vi "_API_BINANCE_POST_DisableFastWithdrawSwich.vi"(0 "BinanceAPI in":refnum<class "BinanceAPI_.lvclass">, 11 "error in (no error)":errorcluster) -> (4 "BinanceAPI out":refnum<class "BinanceAPI_.lvclass">, 14 "Body":string, 15 "error out":errorcluster)   [LabVIEW 2022 SP3, in "BinanceAPI_.lvclass"]
doc: "https://binance-docs.github.io/apidocs/spot/en/#disable-fast-withdraw-switch-user_data"
uses:
  BinanceAPI_.lvclass
  BinanceAPI_.lvclass/BinanceAPI_.ctl
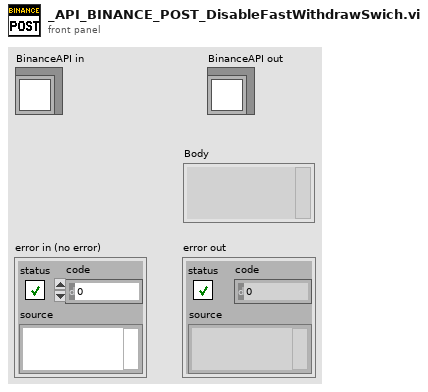
[diagram p1: front panel]
types:
  T1 = enum16{"SPOT", "USDT_FUTURES", "COIN_FUTURES", "VANILLA"}
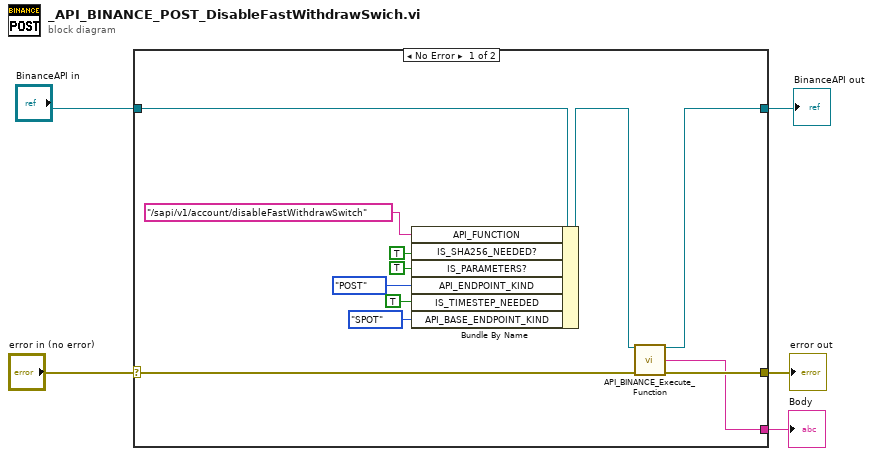
[diagram p0: block diagram]
diagram:
  n1 = case shown="No Error" "error in (no error)" {
    selector: "error in (no error)" -> [w9 w19]
    tunnel: [w8 w19] -> w4
    tunnel: [w10 w18] -> w2
    tunnel: "BinanceAPI in" -> [w13 w18]
    tunnel: [w6 _] -> w1
    frame No Error {
      n2 = Bundle By Name(cluster=w13, "API_FUNCTION"="/sapi/v1/account/disableFastWithdrawSwitch", "IS_SHA256_NEEDED?"=TRUE, "IS_PARAMETERS?"=TRUE, "API_ENDPOINT_KIND"=enum16{"POST", "DELETE", "GET", "PUT"}."POST", "IS_TIMESTEP_NEEDED"=TRUE ("IS_SHA256_NEEDED?"), "API_BASE_ENDPOINT_KIND"=T1."SPOT") -> (w11:refnum<class "BinanceAPI_.lvclass">)
      n3 = call "API_BINANCE_Execute_Function.vi"("BinanceAPI in"=w11, "error in (no error)"=w9) -> ("BinanceAPI out"=w10:refnum<class "BinanceAPI_.lvclass">, "Body"=w6:string, "error out"=w8:errorcluster)  [unwired: 9 in, 2 out]
    }
    frame Error {
    }
  }
  "error out" <- w4
  "BinanceAPI out" <- w2
  "Body" <- w1
